vi "RichToFlatAcquisition_Stream_Data.vi"(5 "OutputClusterType":T1, 11 "InputCluster":T2) -> (3 "OutputCluster":T1)   [LabVIEW 2021, in "Stream_client.lvlib"]
uses:
  Acquisition_Stream_Data.ctl
  Acquisition_Stream_Data_Flat.ctl
  Stream_client.lvlib
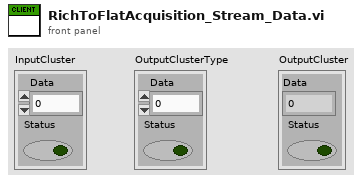
[diagram p1: front panel]
types:
  T1 = typedef "Stream_client.lvlib/Acquisition_Stream_Data_Flat.ctl" = cluster{"Data":i32, "Status":bool}
  T2 = typedef "Stream_client.lvlib/Acquisition_Stream_Data.ctl" = cluster{"Data":i32, "Status":bool}
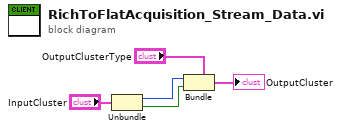
[diagram p0: block diagram]
diagram:
  n1 = Unbundle "Unbundle"("InputCluster") -> ("Data"=w2:i32, "Status"=w1:bool)
  n2 = Bundle "Bundle"(cluster="OutputClusterType", "Data"=w2, "Status"=w1) -> (→"OutputCluster":T1)
